vi "editscenario Load Templates.vi"(7 "Template Keys (empty)":T1, 8 "error in (no error)":errorcluster, 11 "Connection Refnum":T2) -> (0 "error out":errorcluster, 3 "Connection Refnum":T2, 5 "Template Keys":T1)   [LabVIEW 2011]
uses:
  SI.LIB/ODBC/SQL Controls/Connection Refnum.ctl
  Addons/internet/utils/keyedarr.llb/Keyed Array.ctl
  Addons/internet/utils/strutil.llb/Case Matching.ctl
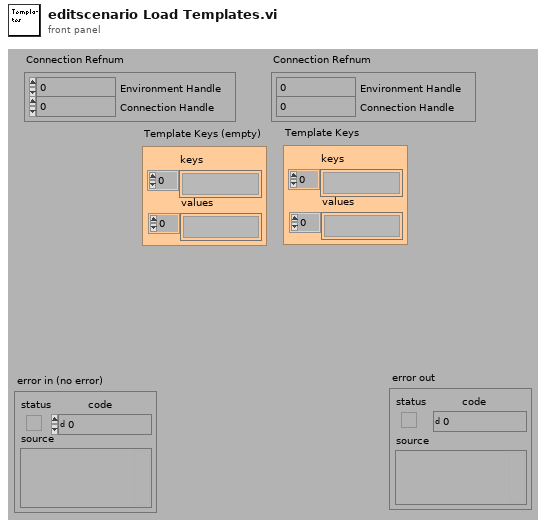
[diagram p1: front panel]
types:
  T1 = typedef "Keyed Array.ctl" = cluster{"keys":string[], "values":string[]}
  T2 = typedef "Connection Refnum.ctl" = cluster{"Environment Handle":i32, "Connection Handle":i32}
  T3 = typedef "Case Matching.ctl" = enum16{"a != A", "a == A", "system"}
  T4 = typedef "Template Record.ctl" = cluster{"ixTemplate":i32, "sxTemplateId":string, "sDescription":string, "sCreator":string, "tCreationDate":timestamp, "sModifier":string, "tModifiedDate":timestamp, "sType":string, "sStyle":string, "sFormat":string, "dWidth":dbl, "dHeight":dbl, "sFilename":string, "sScript":string, "sLayout":string, "sEditor":string, "sStyleProcess":string}
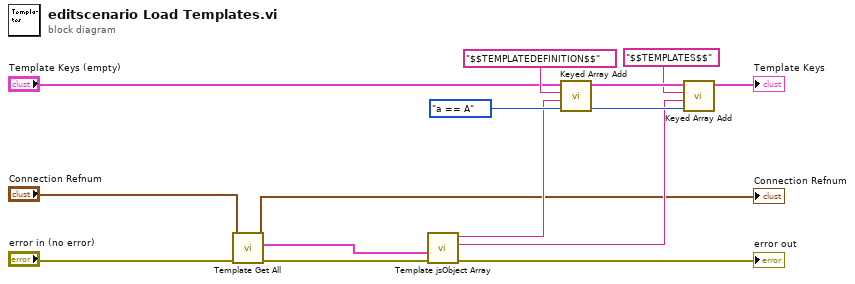
[diagram p0: block diagram]
diagram:
  w9 = Case_Matching."a == A" ("case matching (sensitive)")
  n1 = call "Template Get All.vi"("error in (no error)"="error in (no error)", "Connection Refnum"="Connection Refnum") -> ("error out"=w4:errorcluster, "Templates"=w3:T4[], "Connection Refnum"=→"Connection Refnum":T2)  [unwired: 1 in, 6 out]
  n2 = call "Template jsObject Array.vi"("error in (no error)"=w4, "TEMPLATES (none)"=w3) -> ("error out"=→"error out":errorcluster, "Templates jsObject Array"=w6:string, "Template jsObject Definition"=w7:string)  [unwired: 2 in, 5 out]
  n3 = call "Keyed Array Add.vi"("case matching (sensitive)"=w9, "value"=w7, "key"="$$TEMPLATEDEFINITION$$", "array in"="Template Keys (empty)") -> ("array out"=w13:T1)  [unwired: 3 out]
  n4 = call "Keyed Array Add.vi"("case matching (sensitive)"=w9, "value"=w6, "key"="$$TEMPLATES$$", "array in"=w13) -> ("array out"=→"Template Keys":T1)  [unwired: 3 out]
